vi "Pre Launch Init.vi"(11 "Log in":refnum<class "Log.lvclass"> caption="操作者输入") -> (0 "error out":errorcluster caption="错误输出", 3 "Log out":refnum<class "Log.lvclass"> caption="操作者输出")   [LabVIEW 2018, in "Log.lvlib" / "Log.lvclass"]
doc: "(<B>文件名</B>: Actor Framework.lvlib:Actor.lvclass:Pre Launch Init.vi)\n\n定义启动嵌套操作者方法被调用之后、操作者核心方法开始运行之前的操作。\n\n默认情况下，该方法不执行任何操作。子孙类重写该方法定义具体的操作。"
uses:
  Log.lvclass
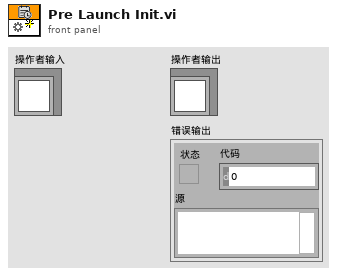
[diagram p1: front panel]
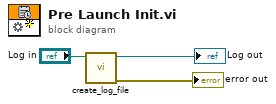
[diagram p0: block diagram]
diagram:
  n1 = call "create_log_file.vi"("Log 输入"="Log in") -> ("error out"=→"error out":errorcluster, "Log 输出"=→"Log out":refnum<class "Log.lvclass">)  [unwired: 9 in]
